vi "HSDIO_6541_Wfm_Script_Load.vi"(7 "Script text":string, 8 "error  in":errorcluster caption="error in", 9 "Table of Waveforms":string[](array[string]), 10 "Timing Waveforms Path":path=path "D:/PIRENEA/TIMING_WFMS", 11 "instrument handle in":refnum<k15>="Sequencer") -> (0 "error out":errorcluster, 2 "FIFO percent used":dbl, 3 "instrument handle out":refnum<k15>)   [LabVIEW 2015]
doc: "This VI demonstrates how to load dynamic waveforms into the board.\n\n1. The waveform binary files are read one by one from the waveform folder.\n2. The data are converted to U32 format and loaded into the on-board memory.\n\nThis VI returns the max memory size of the board, the memory used after loading, and a list of the waveforms loaded. No check of memory overflow is done."
uses:
  <instrlib>/niHSDIO/niHSDIO.llb/niHSDIO Write Named Waveform (1D U32).vi
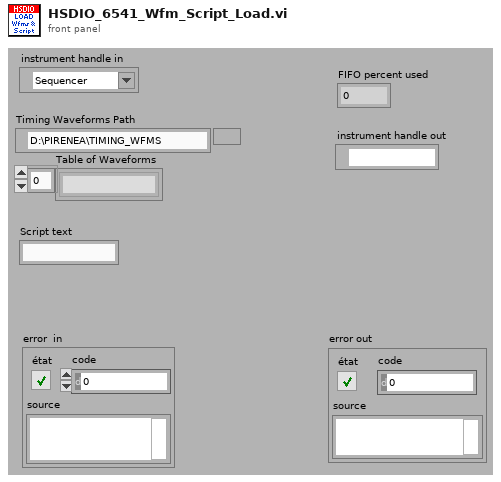
[diagram p1: front panel]
types:
  T1 = enum16{"big-endian, network order", "native, host order", "little-endian"}
  T2 = enum16{"open", "replace", "create", "open or create", "replace or create", "replace or create with confirmation"}
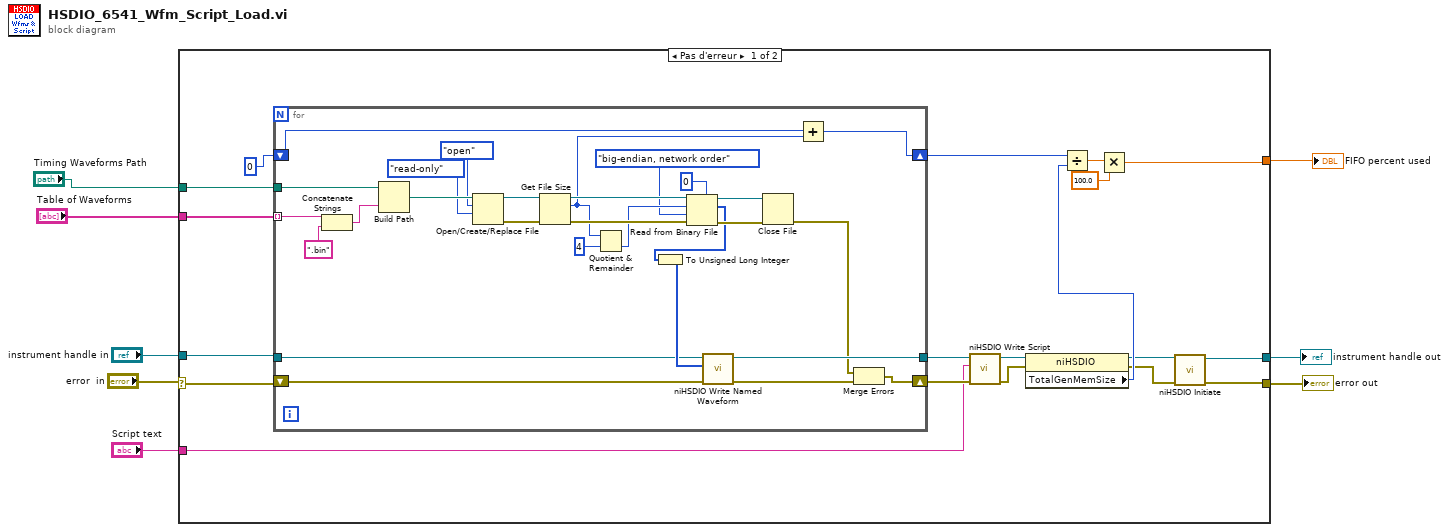
[diagram p0: block diagram]
diagram:
  n1 = case shown="Pas d'erreur" "error  in" {
    selector: "error  in" -> [w26 w56]
    tunnel: [w14 w56] -> w8
    tunnel: [w12 w57] -> w7
    tunnel: "instrument handle in" -> [w27 w57]
    tunnel: [w16 _] -> w4
    tunnel: "Table of Waveforms" -> [w11 _]
    tunnel: "Timing Waveforms Path" -> [w10 _]
    tunnel: "Script text" -> [w9 _]
    frame No Error {
      n2 = for {
        shift-right: [w32] -> w22
        shift-left: w26 -> [w40]
        tunnel: w27 -> [w39]
        tunnel: [w38] -> w24
        shift-right: [w36] -> w20
        shift-left: i64 0 -> [w35]
        tunnel: w11 -> [w29] mode=indexing
        tunnel: w10 -> [w28]
        n3 = Concatenate Strings(w29, ".bin" ("chaîne")) -> (w30:string)
        n4 = Build Path(base path=w28, name or relative path=w30) -> (appended path=w53:path)
        n5 = Open/Create/Replace File(file path (use dialog)=w53, operation (0:open)=T2."open", access (0:read/write)=enum16{"read/write", "read-only", "write-only"}."read-only") -> (refnum out=w55:refnum<file>, error out=w54:errorcluster)  [unwired: 3 in, 1 out]
        n6 = Get File Size(file=w55, error in=w54) -> (refnum out=w49:refnum<file>, size (in bytes)=w37:i64, 0:w47:errorcluster)
        n7 = Quotient & Remainder(x=w37, y=i64 4 ("type size (bytes)")) -> (floor(x/y)=w45:i64)  [unwired: 1 out]
        n8 = Read from Binary File(5:0 ("data type"), 8:w47, 9:T1."big-endian, network order" ("ordre des octets (0 : big-Endian, network order)"), 10:w45, 11:w49) -> (0:w46:errorcluster, 2:w42:i32[], 3:w48:refnum<file>)  [unwired: 1 in, 1 out]
        n9 = To Unsigned Long Integer(number=w42) -> (unsigned 32bit integer=w44:u32[])
        n10 = call-poly <instrlib>:"niHSDIO Write Named Waveform.vi"("error in (no error)"=w40, "data"=w44, "instrument handle"=w39) -> ("error out"=w33:errorcluster, "instrument handle out"=w38:refnum<k15>)  [unwired: 7 in]
        n11 = Close File(refnum=w48, error in=w46) -> (error out=w34:errorcluster)  [unwired: 1 out]
        n12 = Add(x=w35, y=w37) -> (x+y=w36:i64)
        n13 = Merge Errors(w34, w33) -> (w32:errorcluster)
      }
      n14 = call <instrlib>:"niHSDIO Write Script.vi"("error in (no error)"=w22, "script"=w9, "instrument handle"=w24) -> ("error out"=w21:errorcluster, "instrument handle out"=w23:refnum<k15>)  [unwired: 7 in]
      n15 = property on="Property Node" class="niHSDIO"(reference=w23, error in=w21) -> (reference out=w13:refnum<k15>, error out=w15:errorcluster, "TotalGenMemSize"=w19:i32)
      n16 = Divide(x=w20, y=w19) -> (x/y=w18:dbl)
      n17 = Multiply(x=w18, y=100.0) -> (x*y=w16:dbl)
      n18 = call <instrlib>:"niHSDIO Initiate.vi"("error in (no error)"=w15, "instrument handle"=w13) -> ("error out"=w14:errorcluster, "instrument handle out"=w12:refnum<k15>)  [unwired: 8 in]
    }
    frame Error {
    }
  }
  "error out" <- w8
  "instrument handle out" <- w7
  "FIFO percent used" <- w4
